vi "Setpoint2.vi"(8 "ZENONE.Q_set [kVAr]":dbl, 9 "ZENONE.P_set [kW]":dbl, 11 "setpoints IN":dbl[](array[numeric])) -> (2 "OUT":T1)   [LabVIEW 2021]
uses:
  Setpoints_CDA2.ctl
  Setpoints_CDA_ZENONE.ctl
  Setpoints_CDA.ctl
panel:
  # "PV Curtail [%]"
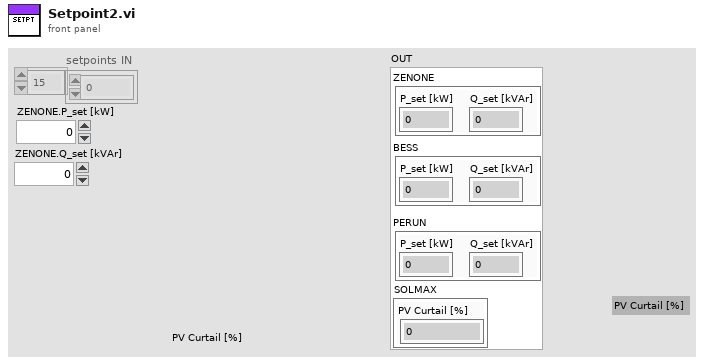
[diagram p1: front panel]
types:
  T1 = typedef "Setpoints_CDA2.ctl" = cluster{"ZENONE":T2, "BESS":T2, "PERUN":T2, "SOLMAX":cluster{"PV Curtail [%]":dbl}}
  T2 = typedef "Setpoints_CDA_ZENONE.ctl" = cluster{"P_set [kW]":dbl, "Q_set [kVAr]":dbl}
  T3 = typedef "Setpoints_CDA.ctl" = cluster{"ZENONE":T2, "BESS":T2, "PERUN":T2, "SOLMAX":T2}
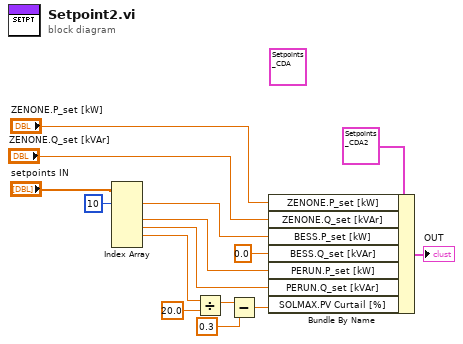
[diagram p0: block diagram]
diagram:
  (unwired) T3 {"ZENONE"={"P_set [kW]"=0.0, "Q_set [kVAr]"=0.0}, "BESS"={"P_set [kW]"=0.0, "Q_set [kVAr]"=0.0}, "PERUN"={"P_set [kW]"=0.0, "Q_set [kVAr]"=0.0}, "SOLMAX"={"P_set [kW]"=0.0, "Q_set [kVAr]"=0.0}} ("CDA_setpoints")
  n1 = Index Array(array="setpoints IN", index #1=10 ("index")) -> (element #1=w12:dbl, element #3=w11:dbl, element #4=w10:dbl, element #5=w6:dbl)  [unwired: 5 in, 2 out]
  n2 = Divide(x=w6, y=20.0) -> (x/y=w4:dbl)
  n3 = Subtract(x=w4, y=0.3) -> (x-y=w3:dbl)
  n4 = Bundle By Name(cluster=T1 {"ZENONE"={"P_set [kW]"=0.0, "Q_set [kVAr]"=0.0}, "BESS"={"P_set [kW]"=0.0, "Q_set [kVAr]"=0.0}, "PERUN"={"P_set [kW]"=0.0, "Q_set [kVAr]"=0.0}, "SOLMAX"={"PV Curtail [%]"=0.0}} ("CDA_setpoints"), "ZENONE.P_set [kW]"="ZENONE.P_set [kW]", "ZENONE.Q_set [kVAr]"="ZENONE.Q_set [kVAr]", "BESS.P_set [kW]"=w12, "BESS.Q_set [kVAr]"=0.0 ("BESS.Q_set"), "PERUN.P_set [kW]"=w11, "PERUN.Q_set [kVAr]"=w10, "SOLMAX.PV Curtail [%]"=w3) -> (→"OUT":T1)
